vi "Shared Variables CD 2.0 RT Driver VI.vi"(7 "Operation":T1, 11 "Device Reference in":T2 format="%.0x") -> (0 "Error Code":i32)   [LabVIEW 2017, in "Shared Variables CD 2.0 Engine.lvlib"]
uses:
  Shared Variables CD 2.0 Engine.lvlib
  <vilib>/NI Veristand/Custom Device API/Custom Device Item Ref.ctl
  <vilib>/NI Veristand/Custom Device API/Hardware Interface Driver VI Operation.ctl
  <vilib>/NI Veristand/Custom Device API/Block Data Reference.ctl
  <vilib>/NI Veristand/Custom Device API/Data Reference.ctl
  Shared DataTypes/SV Process Data.ctl
  Shared DataTypes/URLs.ctl
  <vilib>/NI Veristand/Custom Device API/Data Access Type.ctl
  Shared/Shared Variables CD 2.0 GUID Lookup.vi
  <vilib>/NI Veristand/Custom Device API/Global Data Refs.vi
  <vilib>/NI VeriStand/Custom Device API/Custom Device API.lvlib
  <vilib>/NI Veristand/Custom Device Tools/Custom Device Utility Library/Custom Device Utility Library.lvlib
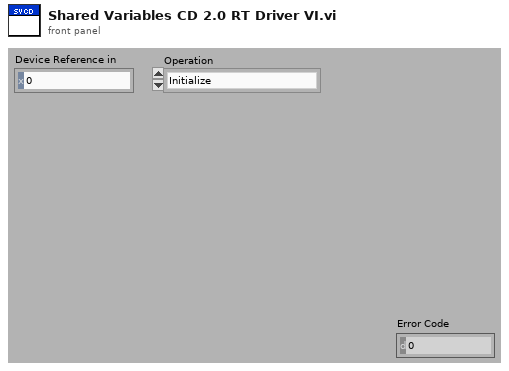
[diagram p1: front panel]
types:
  T1 = typedef "Custom Device API.lvlib/Hardware Interface Driver VI Operation.ctl" = enum16{"Initialize", "Start", "Read Data from HW", "Write Data to HW", "Close"}
  T2 = typedef "Custom Device API.lvlib/Custom Device Item Ref.ctl" = u64
  T3 = typedef "Custom Device API.lvlib/Block Data Reference.ctl" = cluster{"Data Reference":T4, "Offset":u64, "Length":u64}
  T4 = typedef "Custom Device API.lvlib/Data Reference.ctl" = i32
  T5 = typedef "SV Process Data.ctl" = cluster{"Write URLs":T6, "Read URLs":T6, "Write SV FIFO":string, "Read SV FIFO":string, "Status Notifier":string, "Update Rate":u32}
  T6 = typedef "URLs.ctl" = cluster{"URLs":string[], "Index DBL":i32[], "Index Bool":i32[]}
  T7 = cluster{"Output Ref":cluster{"Block Data Refs":T3[], "Values Array":dbl[]}, "Input Ref":cluster{"Block Data Refs":T3[], "Values Array":dbl[]}, "Write FIFO":refnum<k33>, "Read FIFO":refnum<k33>, "Status":refnum<notifier>, "Process Data":T5, "Device Error":errorcluster}
  T8 = typedef "Custom Device API.lvlib/Data Access Type.ctl" = enum16{"Read", "Write"}
  T9 = cluster{"Block Data Refs":T3[], "Values Array":dbl[]}
  T10 = typedef "Custom Device API.lvlib/Custom Device Target Type.ctl" = enum16{"PharLap", "VxWorks", "Windows", "Linux_32_ARM", "Linux_x64"}
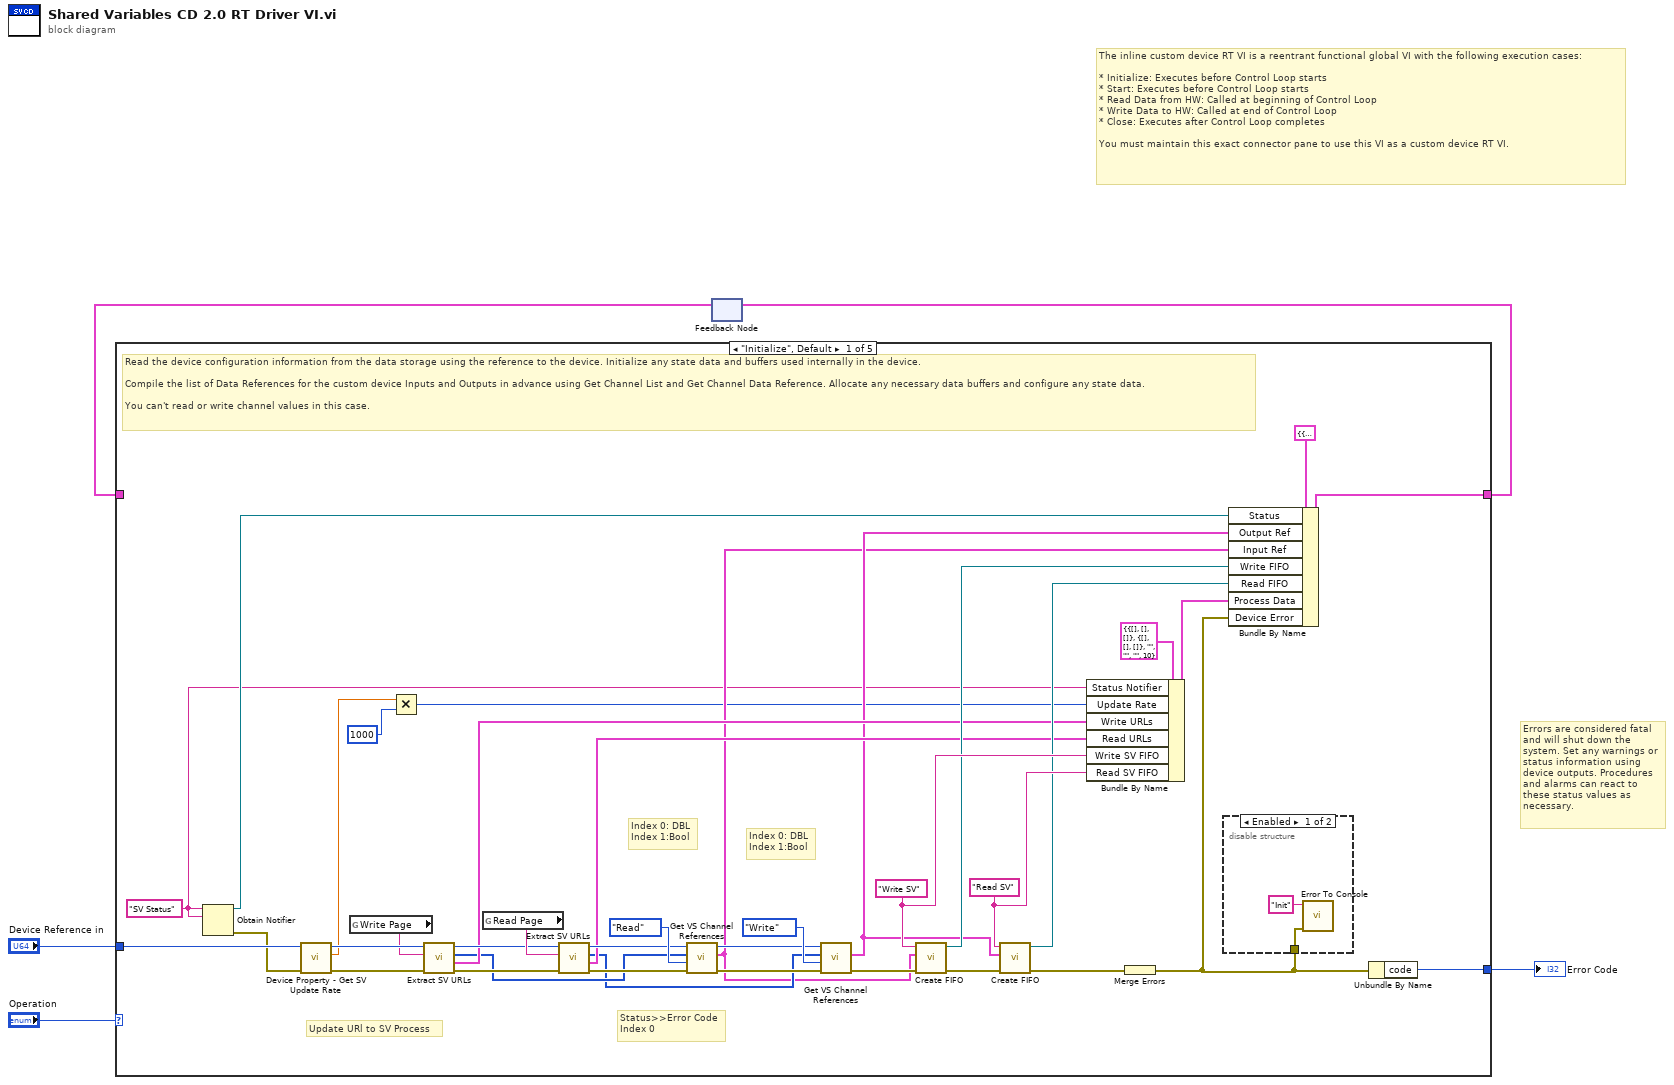
[diagram p0: block diagram]
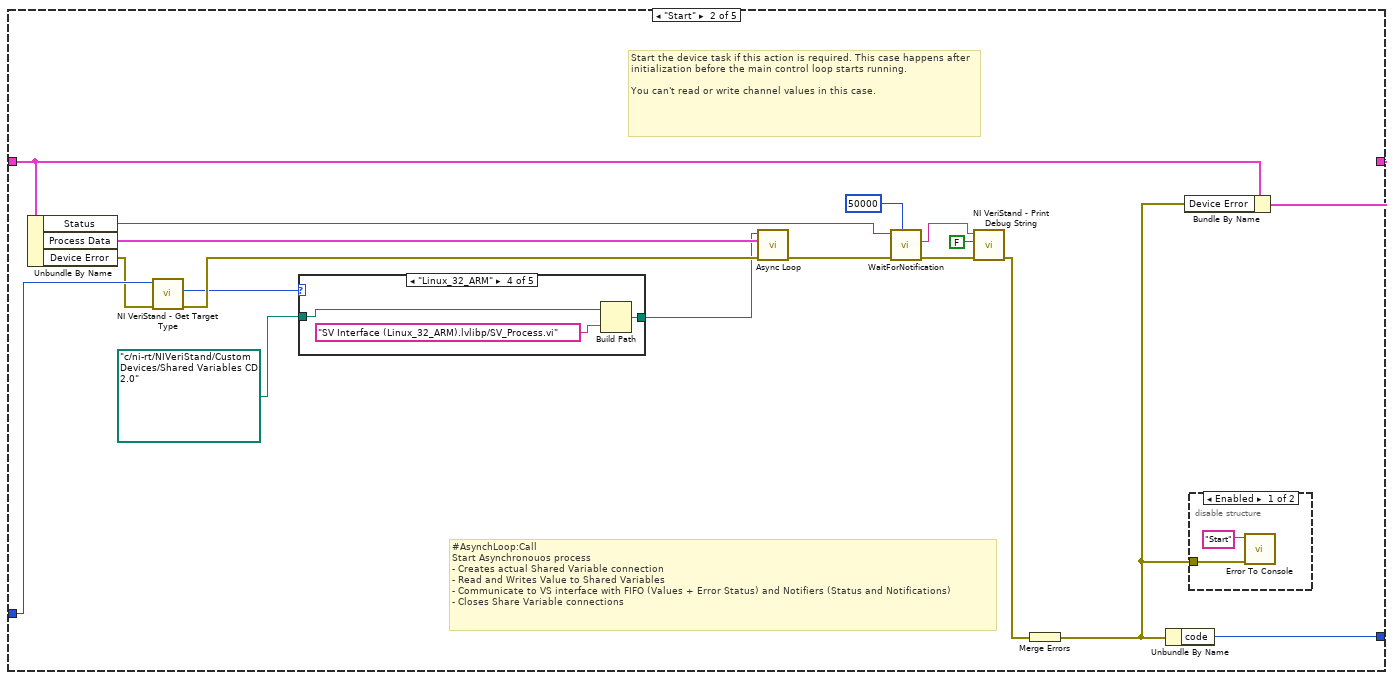
[diagram p3: hidden frame]
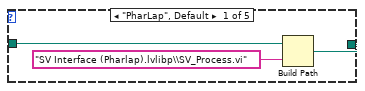
[diagram p4: hidden frame]
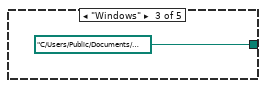
[diagram p6: hidden frame]
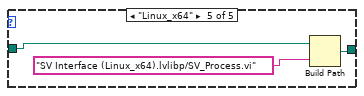
[diagram p7: hidden frame]
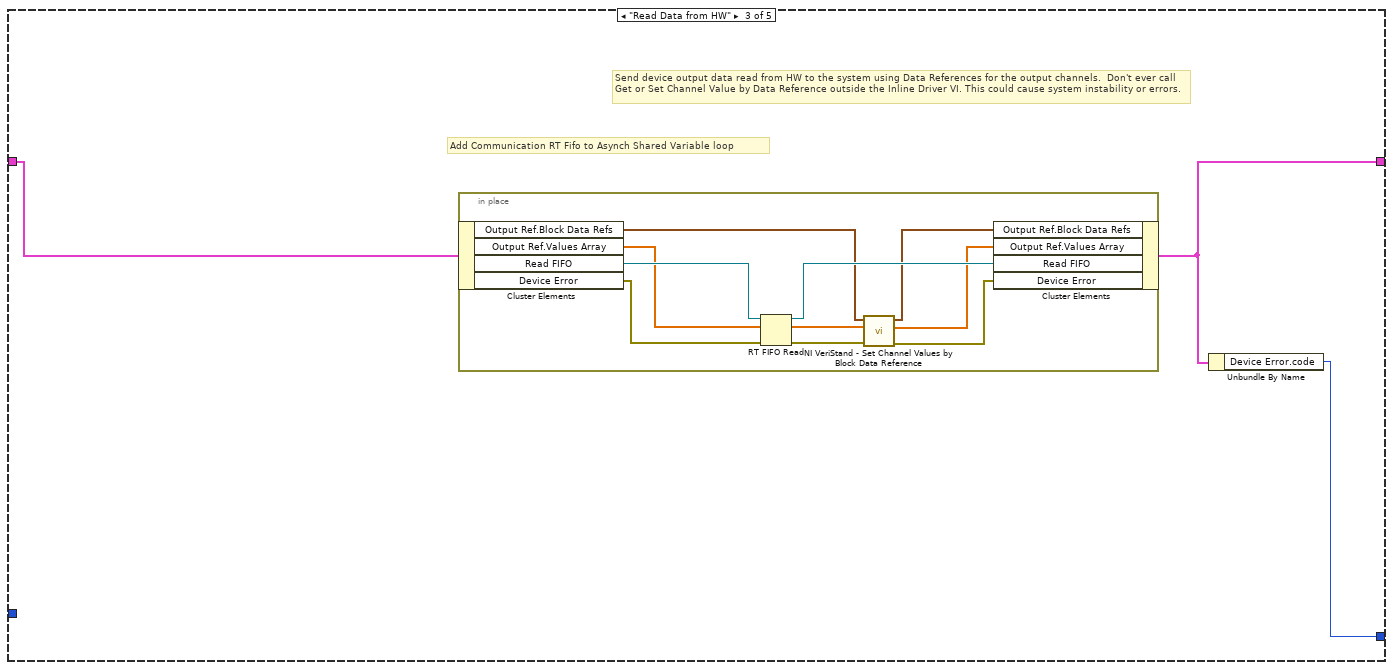
[diagram p9: hidden frame]
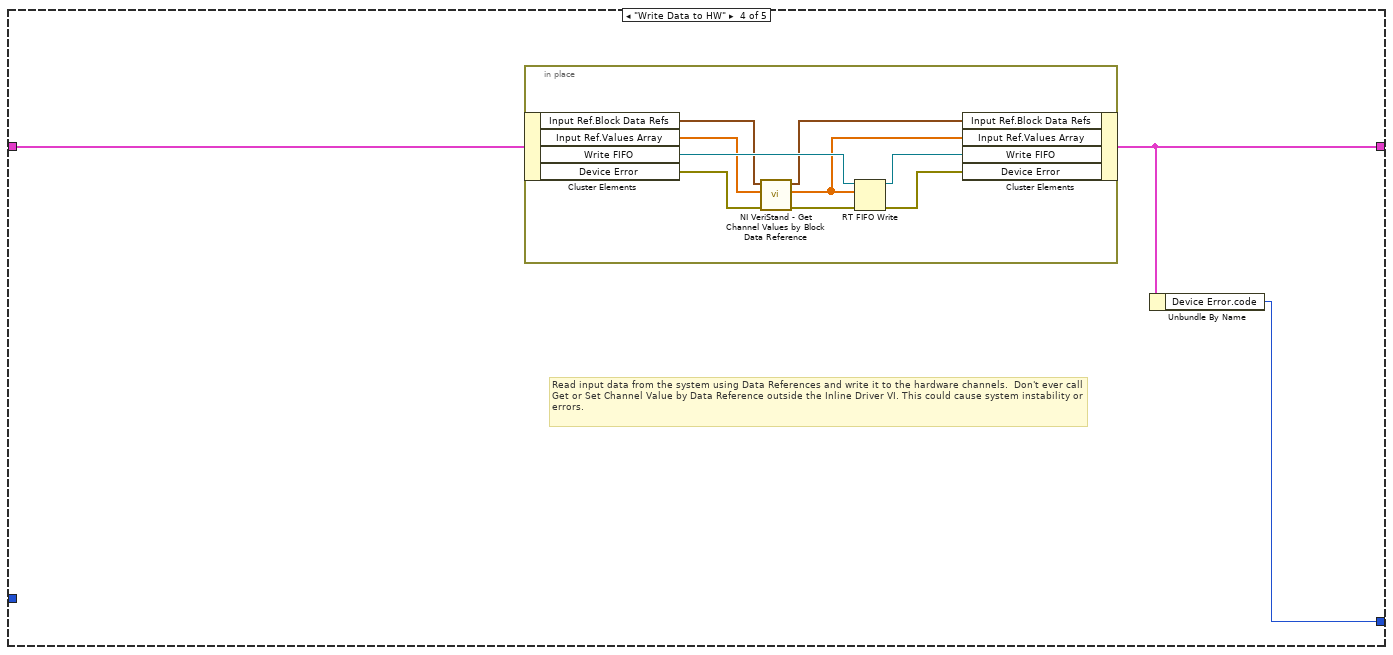
[diagram p10: hidden frame]
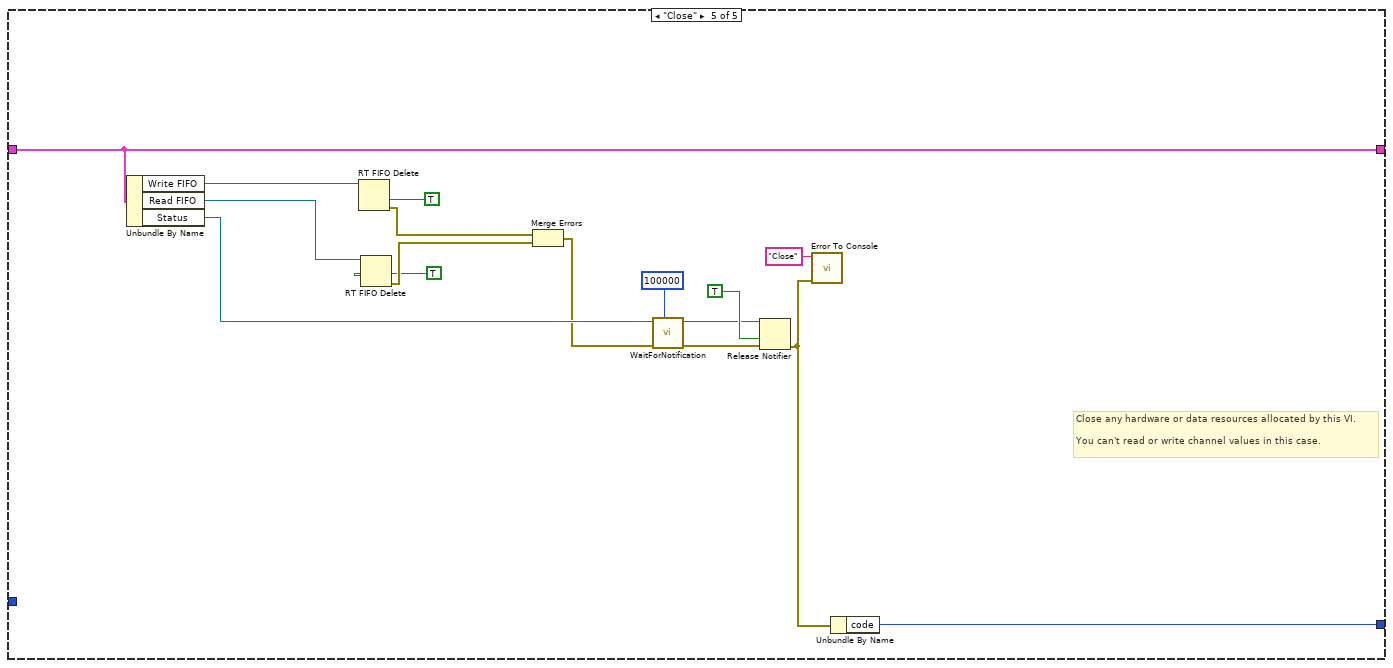
[diagram p11: hidden frame]
diagram:
  # "Errors are considered fatal and will shut down the system. Set any warnings or status information using device outputs. Procedures and alarms can react to these status values as necessary."
  # "The inline custom device RT VI is a reentrant functional global VI with the following execution cases:\n\n* Initialize: Executes before Control Loop starts\n* Start: Executes before Control Loop starts\n* Read Data from HW: Called at beginning of Control Loop\n* Write Data to HW: Called at end of Control Loop\n* Close: Executes after Control Loop completes\n\nYou must maintain this exact connector pane to use this VI as a custom device RT VI."
  n1 = feedback #1() -> (w3:T7)  [unwired: 1 out]
  n2 = case shown="\"Initialize\", Default" "Operation" {
    tunnel: [w43 w62 w78 w91 w116] -> w4
    tunnel: w3 -> [_ w53 w79 w92 w116]
    tunnel: "Device Reference in" -> [w32 w51 _ _ _]
    tunnel: [w41 w63 w77 w90 w117] -> w1
    frame "Initialize", Default {
      w9 = "SV Status" ("name (unnamed)")
      w22 = "Write SV" ("FIFO Name")
      w23 = "Read SV" ("name (unnamed)")
      # "Update URl to SV Process"
      # "Index 0: DBL\nIndex 1:Bool"
      # "Index 0: DBL\nIndex 1:Bool"
      # "Status>>Error Code\nIndex 0"
      # "Read the device configuration information from the data storage using the reference to the device. Initialize any state data and buffers used internally in the device.\n\nCompile the list of Data References for the custom device Inputs and Outputs in advance using Get Channel List and Get Channel Data Reference. Allocate any necessary data buffers and configure any state data.\n\nYou can't read or write channel values in this case."
      n3 = Obtain Notifier(name (unnamed)=w9, notification data type=w9) -> (notifier out=w34:refnum<notifier>, error out=w30:errorcluster)  [unwired: 2 in, 1 out]
      n4 = call "Device Property - Get SV Update Rate.vi"("error in (no error)"=w30, "Device Ref in"=w32) -> ("error out"=w29:errorcluster, "Update Rate (ms)"=w8:dbl, "Device Ref out"=w31:T2)  [unwired: 7 in]
      n5 = global read "Shared Variables CD 2.0 GUID Lookup.vi" "Write Page"() -> (w18:string)
      n6 = Multiply(x=w8, y=u32 1000) -> (x*y=w7:u32)
      n7 = call "Extract SV URLs.vi"("error in (no error)"=w29, "Page"=w18, "Device Reference in"=w31) -> ("error out"=w16:errorcluster, "SV"=w15:T6, "Channel Refs"=w14:T2[], "Device Reference out"=w17:T2)  [unwired: 5 in]
      n8 = global read "Shared Variables CD 2.0 GUID Lookup.vi" "Read Page"() -> (w19:string)
      n9 = call "Extract SV URLs.vi"("error in (no error)"=w16, "Page"=w19, "Device Reference in"=w17) -> ("error out"=w36:errorcluster, "SV"=w13:T6, "Channel Refs"=w12:T2[], "Device Reference out"=w35:T2)  [unwired: 5 in]
      n10 = call "Get VS Channel References.vi"("error in (no error)"=w36, "Access (Read)"=Data_Access_Type."Read" ("Access"), "Channel Refs"=w14, "Device Reference in"=w35) -> ("error out"=w38:errorcluster, "DataRef"=w10:T9, "Device Reference out"=w39:T2)  [unwired: 5 in]
      n11 = call "Get VS Channel References.vi"("error in (no error)"=w38, "Access (Read)"=Data_Access_Type."Write" ("Access"), "Channel Refs"=w12, "Device Reference in"=w39) -> ("error out"=w26:errorcluster, "DataRef"=w11:T9)  [unwired: 5 in, 1 out]
      n12 = call "Create FIFO.vi"("error in (no error)"=w26, "DataRef"=w10, "FIFO Name"=w22) -> ("error out"=w25:errorcluster, "FIFO Ref"=w20:refnum<k33>)  [unwired: 7 in]
      n13 = call "Create FIFO.vi"("error in (no error)"=w25, "DataRef"=w11, "FIFO Name"=w23) -> ("error out"=w24:errorcluster, "FIFO Ref"=w21:refnum<k33>)  [unwired: 7 in]
      n14 = Bundle By Name(cluster=T5 {"Write URLs"={"URLs"=[], "Index DBL"=[], "Index Bool"=[]}, "Read URLs"={"URLs"=[], "Index DBL"=[], "Index Bool"=[]}, "Write SV FIFO"="", "Read SV FIFO"="", "Status Notifier"="", "Update Rate"=10} ("Cluster"), "Status Notifier"=w9, "Update Rate"=w7, "Write URLs"=w15, "Read URLs"=w13, "Write SV FIFO"=w22, "Read SV FIFO"=w23) -> (w27:T5)
      n15 = Merge Errors(w24) -> (w33:errorcluster)
      n16 = disable-structure shown="Enabled" {
        disable-tunnel: w33 -> [w45 _]
        frame Enabled {
          n17 = call "Error To Console.vi"("error in (no error)"=w45, "Add Text to Message"="Init") -> ()  [unwired: 10 in]
        }
        frame Disabled {
        }
      }
      n18 = Bundle By Name(cluster=T7 {"Output Ref"={"Block Data Refs"=[], "Values Array"=[]}, "Input Ref"={"Block Data Refs"=[], "Values Array"=[]}, "Write FIFO"=refnum, "Read FIFO"=refnum, "Status"=refnum, "Process Data"={"Write URLs"={"URLs"=[], "Index DBL"=[], "Index Bool"=[]}, "Read URLs"={"URLs"=[], "Index DBL"=[], "Index Bool"=[]}, "Write SV FIFO"="", "Read SV FIFO"="", "Status Notifier"="", "Update Rate"=10}, "Device Error"={"status"=FALSE, "code"=0, "source"=""}}, "Status"=w34, "Output Ref"=w11, "Input Ref"=w10, "Write FIFO"=w20, "Read FIFO"=w21, "Process Data"=w27, "Device Error"=w33) -> (w43:T7)
      n19 = Unbundle By Name(w33) -> ("code"=w41:i32)
    }
    frame "Start" {
      # "#AsynchLoop:Call\nStart Asynchronouos process\n- Creates actual Shared Variable connection\n- Read and Writes Value to Shared Variables\n- Communicate to VS interface with FIFO (Values + Error Status) and Notifiers (Status and Notifications)\n- Closes Share Variable connections"
      # "Start the device task if this action is required. This case happens after initialization before the main control loop starts running.\n\nYou can't read or write channel values in this case."
      n20 = Unbundle By Name(w53) -> ("Status"=w61:refnum<notifier>, "Process Data"=w54:T5, "Device Error"=w50:errorcluster)
      n21 = call <vilib>:"NI VeriStand - Get Target Type.vi"("error in (no error)"=w50, "Item Ref in"=w51) -> ("error out"=w49:errorcluster, "Target Type"=w47:T10)  [unwired: 7 in, 1 out]
      n22 = case shown="\"Linux_32_ARM\"" w47 {
        tunnel: path "c:/ni-rt/NIVeriStand/Custom Devices/Shared Variables CD 2.0" -> [w65 w67 _ w71 w73]
        tunnel: [w64 w67 path "C:/Users/Public/Documents/National Instruments/NI VeriStand 2016/Custom Devices/Shared Variables CD 2.0/Data/SV Interface (Pharlap).lvlibp/SV_Process.vi" w70 w72] -> w46
        frame "PharLap", Default {
          n23 = Build Path(base path=w65, name or relative path="SV Interface (Pharlap).lvlibp\\SV_Process.vi") -> (appended path=w64:path)
        }
        frame "VxWorks" {
        }
        frame "Windows" {
        }
        frame "Linux_32_ARM" {
          n24 = Build Path(base path=w71, name or relative path="SV Interface (Linux_32_ARM).lvlibp/SV_Process.vi") -> (appended path=w70:path)
        }
        frame "Linux_x64" {
          n25 = Build Path(base path=w73, name or relative path="SV Interface (Linux_x64).lvlibp/SV_Process.vi") -> (appended path=w72:path)
        }
      }
      n26 = call "Async Loop.vi"("error in (no error)"=w49, "Process Data"=w54, "Path"=w46) -> ("error out"=w55:errorcluster)  [unwired: 8 in]
      n27 = call "WaitForNotification.vi"("timeout in ms (-1)"=50000, "error in (no error)"=w55, "Notifier in"=w61) -> ("error out"=w58:errorcluster, "Status out"=w57:string)  [unwired: 6 in, 1 out]
      n28 = call <vilib>:"NI VeriStand - Print Debug String.vi"("error in (no error)"=w58, "Add to log file? (T)"=FALSE, "Message"=w57) -> ("error out"=w52:errorcluster)  [unwired: 8 in]
      n29 = Merge Errors(w52) -> (w59:errorcluster)
      n30 = Unbundle By Name(w59) -> ("code"=w63:i32)
      n31 = Bundle By Name(cluster=w53, "Device Error"=w59) -> (w62:T7)
      n32 = disable-structure shown="Enabled" {
        disable-tunnel: w59 -> [w76 _]
        frame Enabled {
          n33 = call "Error To Console.vi"("error in (no error)"=w76, "Add Text to Message"="Start") -> ()  [unwired: 10 in]
        }
        frame Disabled {
        }
      }
    }
    frame "Read Data from HW" {
      # "Add Communication RT Fifo to Asynch Shared Variable loop"
      # "Send device output data read from HW to the system using Data References for the output channels.  Don't ever call Get or Set Channel Value by Data Reference outside the Inline Driver VI. This could cause system instability or errors."
      n34 = in-place {
        n35 = in-place-cluster #2(w79) -> ("Output Ref.Block Data Refs"=w81:T3[], "Output Ref.Values Array"=w83:dbl[], "Read FIFO"=w87:refnum<k33>, "Device Error"=w89:errorcluster)
        n36 = RT FIFO Read(0:w87, 1:w83, 3:w89) -> (8:w84:refnum<k33>, 9:w86:dbl[], 11:w85:errorcluster)  [unwired: 1 in, 2 out]
        n37 = call <vilib>:"NI VeriStand - Set Channel Values by Block Data Reference.vi"("error in (no error)"=w85, "Values Array in"=w86, "Block Data Ref"=w81) -> ("error out"=w88:errorcluster, "Values Array out"=w82:dbl[], "Block Data Ref dup"=w80:T3[])  [unwired: 6 in]
        n38 = in-place-cluster #2("Output Ref.Block Data Refs"=w80, "Output Ref.Values Array"=w82, "Read FIFO"=w84, "Device Error"=w88) -> (w78:T7)
      }
      n39 = Unbundle By Name(w78) -> ("Device Error.code"=w77:i32)
    }
    frame "Write Data to HW" {
      # "Read input data from the system using Data References and write it to the hardware channels.  Don't ever call Get or Set Channel Value by Data Reference outside the Inline Driver VI. This could cause system instability or errors."
      n40 = in-place {
        n41 = in-place-cluster #3(w92) -> ("Input Ref.Block Data Refs"=w96:T3[], "Input Ref.Values Array"=w97:dbl[], "Write FIFO"=w98:refnum<k33>, "Device Error"=w101:errorcluster)
        n42 = call <vilib>:"NI VeriStand - Get Channel Values by Block Data Reference.vi"("error in (no error)"=w101, "Values Array in"=w97, "Block Data Ref"=w96) -> ("error out"=w100:errorcluster, "Values Array out"=w94:dbl[], "Block Data Ref dup"=w95:T3[])  [unwired: 6 in]
        n43 = RT FIFO Write(0:w98, 1:w94, 3:w100) -> (8:w93:refnum<k33>, 11:w99:errorcluster)  [unwired: 2 in, 2 out]
        n44 = in-place-cluster #3("Input Ref.Block Data Refs"=w95, "Input Ref.Values Array"=w94, "Write FIFO"=w93, "Device Error"=w99) -> (w91:T7)
      }
      n45 = Unbundle By Name(w91) -> ("Device Error.code"=w90:i32)
    }
    frame "Close" {
      # "Close any hardware or data resources allocated by this VI.\n\nYou can't read or write channel values in this case."
      n46 = Unbundle By Name(w116) -> ("Write FIFO"=w102:refnum<k33>, "Read FIFO"=w104:refnum<k33>, "Status"=w112:refnum<notifier>)
      n47 = RT FIFO Delete(0:w102, 2:TRUE ("force destroy? (F)")) -> (11:w108:errorcluster)  [unwired: 1 in]
      n48 = RT FIFO Delete(0:w104, 2:TRUE ("force destroy? (F)")) -> (11:w107:errorcluster)  [unwired: 1 in]
      n49 = Merge Errors(w108, w107) -> (w106:errorcluster)
      n50 = call "WaitForNotification.vi"("timeout in ms (-1)"=100000, "error in (no error)"=w106, "Notifier in"=w112) -> ("error out"=w110:errorcluster, "Notifier out"=w111:refnum<notifier>)  [unwired: 6 in, 1 out]
      n51 = Release Notifier(notifier=w111, force destroy? (F)=TRUE, error in (no error)=w110) -> (error out=w114:errorcluster)  [unwired: 2 out]
      n52 = call "Error To Console.vi"("error in (no error)"=w114, "Add Text to Message"="Close") -> ()  [unwired: 10 in]
      n53 = Unbundle By Name(w114) -> ("code"=w117:i32)
    }
  }
  "Error Code" <- w1
  n54 = feedback-in #1(w4) -> ()
